vi "Test harness - Is part of vi lib.vi"(11 "Type of file to test":T1=".vi") -> (0 "error out":errorcluster, 3 "Part of vi lib":bool)   [LabVIEW 2021]
uses:
  Test harness file type.ctl
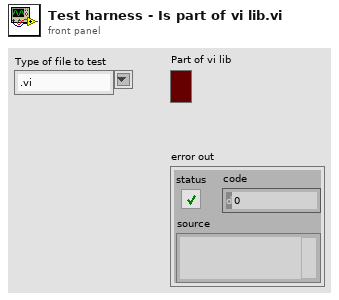
[diagram p1: front panel]
types:
  T1 = typedef "Test harness file type.ctl" = string
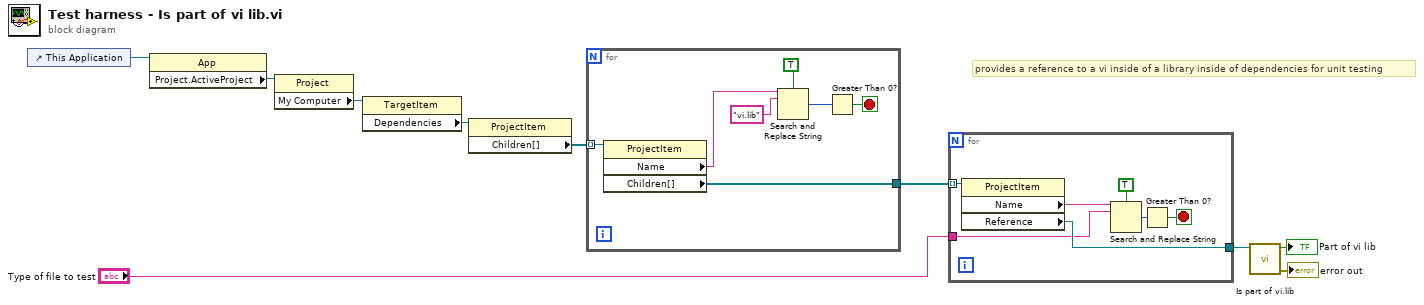
[diagram p0: block diagram]
diagram:
  # "provides a reference to a vi inside of a library inside of dependencies for unit testing"
  n1 = control-ref of="This Application"() -> (w3:refnum<vi>)
  n2 = property class="App"(reference=w3) -> ("Project.ActiveProject"=w10:refnum<vi>)  [unwired: 1 in, 2 out]
  n3 = property class="Project"(reference=w10) -> ("My Computer"=w7:refnum<vi>)  [unwired: 1 in, 2 out]
  n4 = property class="TargetItem"(reference=w7) -> ("Dependencies"=w9:refnum<vi>)  [unwired: 1 in, 2 out]
  n5 = property class="ProjectItem"(reference=w9) -> ("Children[]"=w8:refnum<vi>[])  [unwired: 1 in, 2 out]
  n6 = for {
    tunnel: w8 -> [w17] mode=indexing
    tunnel: [w12] -> w1
    stop <- w16 stop-if-true
    n7 = property class="ProjectItem"(reference=w17) -> ("Name"=w15:string, "Children[]"=w12:refnum<vi>[])  [unwired: 1 in, 2 out]
    n8 = Search and Replace String(case sensitive?=TRUE ("ignore case? (F)"), input string=w15, search string="vi.lib" ("search string/char (-)")) -> (number of replacements=w11:i32)  [unwired: 5 in, 3 out]
    n9 = Greater Than 0?(x=w11) -> (x > 0?=w16:bool)
  }
  n10 = for {
    tunnel: w1 -> [w24] mode=indexing
    tunnel: [w20] -> w6
    tunnel: "Type of file to test" -> [w18]
    stop <- w21 stop-if-true
    n11 = property class="ProjectItem"(reference=w24) -> ("Name"=w22:string, "Reference"=w20:refnum<vi>)  [unwired: 1 in, 2 out]
    n12 = Search and Replace String(case sensitive?=TRUE ("ignore case? (F)"), input string=w22, search string=w18) -> (number of replacements=w19:i32)  [unwired: 5 in, 3 out]
    n13 = Greater Than 0?(x=w19) -> (x > 0?=w21:bool)
  }
  n14 = call "Is part of vi.lib"("VI Reference"=w6) -> ("error out"=→"error out":errorcluster, "Library member part of vi.lib"=→"Part of vi lib":bool)  [unwired: 9 in]
